vi "Set Dilicon Measurement.vi"(8 "error in (no error)":errorcluster, 10 "Dilico Measurement Controls":T2 {"Wait time [ms]" max=26}, 11 "input cluster":T1={"Session_Control"="Sess_Control", "Session_Params"="Sess_Params", "Session_Actuals"="Sess_Actuals", "Session_Acknowledge"="Sess_Ack", "Session_H2_Sensor"="H2_Sensor_Session", "Session_DILICO_MeasurementRequest"="Session_DILICO_MeasurementRequest", "Session_DILICO_Voltages"="Session_DILICO_CELLVoltage"}) -> (0 "error out":errorcluster, 3 "output cluster":T1={"Session_Control"="Session_Control", "Session_Params"="Session_Params", "Session_Actuals"="Session_Actuals", "Session_Acknowledge"="Session_Acknowledge", "Session_H2_Sensor"="H2_Sensor_Session", "Session_DILICO_MeasurementRequest"="Session_DILICO_MeasurementRequest", "Session_DILICO_Voltages"="Session_DILICO_CELLVoltage"})   [LabVIEW 2025, in "phlair-busch-can-bus.lvlib"]
uses:
  phlair-busch-can-bus.lvlib
  DilicoControls.ctl
  CAN Frame Sessions.ctl
  <vilib>/xnet/xnet.llb/XNET Write (Signal Single-point).vi
  <resource>/objmgr/xnet.rc
panel:
  out "Request array":u8[](array[numeric]) format="%.0x"
  out "Array 2":u32[](array[numeric])
  out "Array":dbl[](array[numeric])
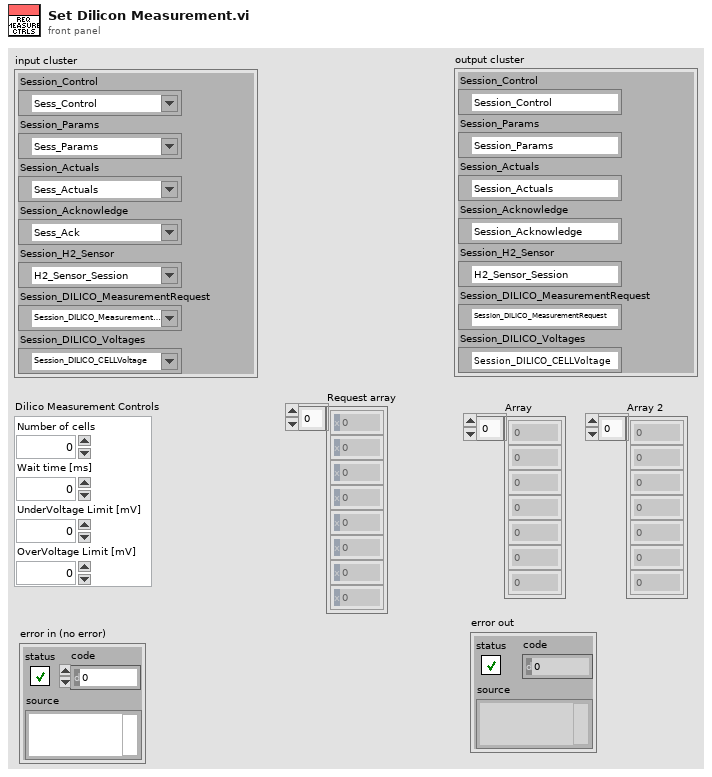
[diagram p1: front panel]
types:
  T1 = typedef "phlair-busch-can-bus.lvlib/CAN Frame Sessions.ctl" = cluster{"Session_Control":refnum<k21>, "Session_Params":refnum<k21>, "Session_Actuals":refnum<k21>, "Session_Acknowledge":refnum<k21>, "Session_H2_Sensor":refnum<k21>, "Session_DILICO_MeasurementRequest":refnum<k21>, "Session_DILICO_Voltages":refnum<k21>}
  T2 = typedef "phlair-busch-can-bus.lvlib/DilicoControls.ctl" = cluster{"Number of cells":u8, "Wait time [ms]":sgl, "UnderVoltage Limit [mV]":u16, "OverVoltage Limit [mV]":u16}
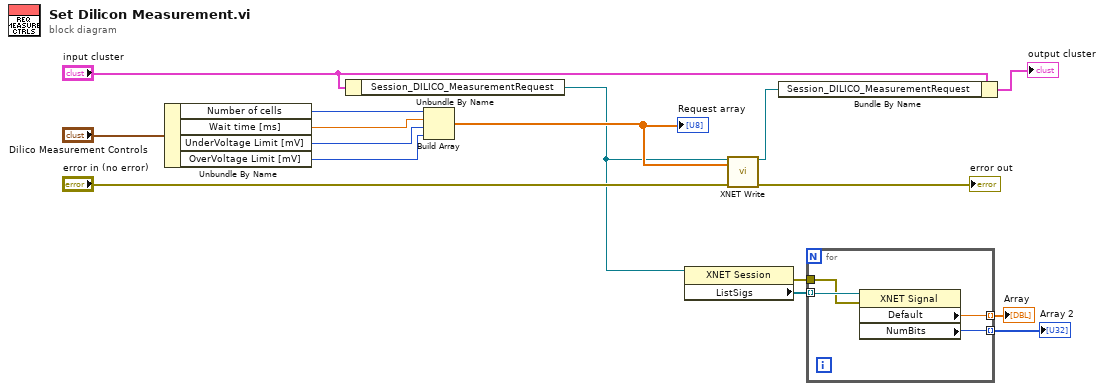
[diagram p0: block diagram]
diagram:
  n1 = Unbundle By Name("Dilico Measurement Controls") -> ("Number of cells"=w13:u8, "Wait time [ms]"=w3:sgl, "UnderVoltage Limit [mV]"=w2:u16, "OverVoltage Limit [mV]"=w1:u16)
  n2 = Unbundle By Name("input cluster") -> ("Session_DILICO_MeasurementRequest"=w4:refnum<k21>)
  n3 = Build Array(w13, w3, w2, w1) -> (w6:sgl[])
  "Request array" <- w6
  n4 = property class="XNET Session"(reference=w4) -> (error out=w7:errorcluster, "ListSigs"=w10:refnum<k21>[])  [unwired: 1 in, 1 out]
  n5 = call-poly <vilib>:"XNET Write.vi"("session in"=w4, "data"=w6, "error in (no error)"="error in (no error)") -> ("session out"=w5:refnum<k21>, "error out"=→"error out":errorcluster)  [unwired: 11 in]
  n6 = Bundle By Name(cluster="input cluster", "Session_DILICO_MeasurementRequest"=w5) -> (→"output cluster":T1)
  n7 = for {
    tunnel: w10 -> [w20] mode=indexing
    tunnel: [w19] -> w9 mode=indexing
    tunnel: [w18] -> w8 mode=indexing
    tunnel: w7 -> [w17]
    n8 = property class="XNET Signal"(reference=w20, error in=w17) -> ("Default"=w19:dbl, "NumBits"=w18:u32)  [unwired: 2 out]
  }
  "Array" <- w9
  "Array 2" <- w8
